vi "RTP.vi"() -> ()   [LabVIEW 2015]
uses:
  <vilib>/myRIO/Common/Instrument Driver Framework/myRIO v1.0/UART/vis/myRIO v1.0 Close UART.vi
  <vilib>/FPGAPlugInAG/myRIO-1900/niLvFpga_Open_myRIO-1900.vi
  <vilib>/rvi/interface/common/dynamic/niFpgaDynamicAddResources.vi
  <vilib>/Utility/error.llb/Error Cluster From Error Code.vi
  <vilib>/rvi/errors/niLvFpgaAdjustHostInterfaceError.vi
  <vilib>/FPGAPlugInAG/Dynamic/niLvFpga_Close_Dynamic.vi
  <vilib>/myRIO/Common/Instrument Driver Framework/Utilities/vis/FPGA Ref Manager.vi
  <vilib>/myRIO/Common/Instrument Driver Framework/myRIO v1.0/myRIO v1.0 Reset FPGA.vi
  <vilib>/myRIO/Common/Instrument Driver Framework/myRIO v1.0/IRQ/vis/myRIO v1.0 IRQ Info FGV.vi
  <vilib>/myRIO/Common/Instrument Driver Framework/myRIO v1.0/IRQ/vis/myRIO v1.0 Timer IRQ Info FGV.vi
  <vilib>/myRIO/Common/Instrument Driver Framework/myRIO v1.0/IRQ/vis/myRIO v1.0 ISR Agent.vi
  <vilib>/rvi/interface/nirviOpenFPGA/nirviOpenFPGA.xnode
  FPGA Bitfiles/adquisicion_FPGATarget_FPGA_kaZO9Kqay0w.lvbitx
  FPGA.vi
  <vilib>/rvi/interface/nirviReadWriteControl/nirviReadWriteControl.xnode
  <vilib>/rvi/interface/nirviCloseFPGA/nirviCloseFPGA.xnode
  <vilib>/rvi/interface/Simulation/niFpgaSimulationCallBeginRW.vi
  <vilib>/myRIO/Instrument Drivers/Utilities/Utilities.lvlib
  NiFpgaLv.dll
panel:
  out "Fedders current":cluster{dbl[], dbl[]}[](graph)
  out "Size":dbl
  out "u2":u16[](graph)
  out "vb":dbl
  out "vB":dbl
  out "ir":dbl
  out "i_3":dbl
  out "1_2":dbl
  out "i_1":dbl
  out "Ring":u16(ring)
  out "d 3":i16[](graph)
  out "d 2":i16[](graph)
  out "d 1":i16[](graph)
  out "i_3":u16[](graph)
  out "v_b":u16[](graph)
  out "v_B":u16[](graph)
  out "i_1":u16[](graph)
  in  "clear":bool
  in  "stop":bool
  out "State RTP":enum16{"inicio", "delay", "pedir", "guardar"}(ring)
  out "State FPGA":T1(ring)
  out "i_2":u16[](graph)
  in  "Get data":bool
  out "Data":string
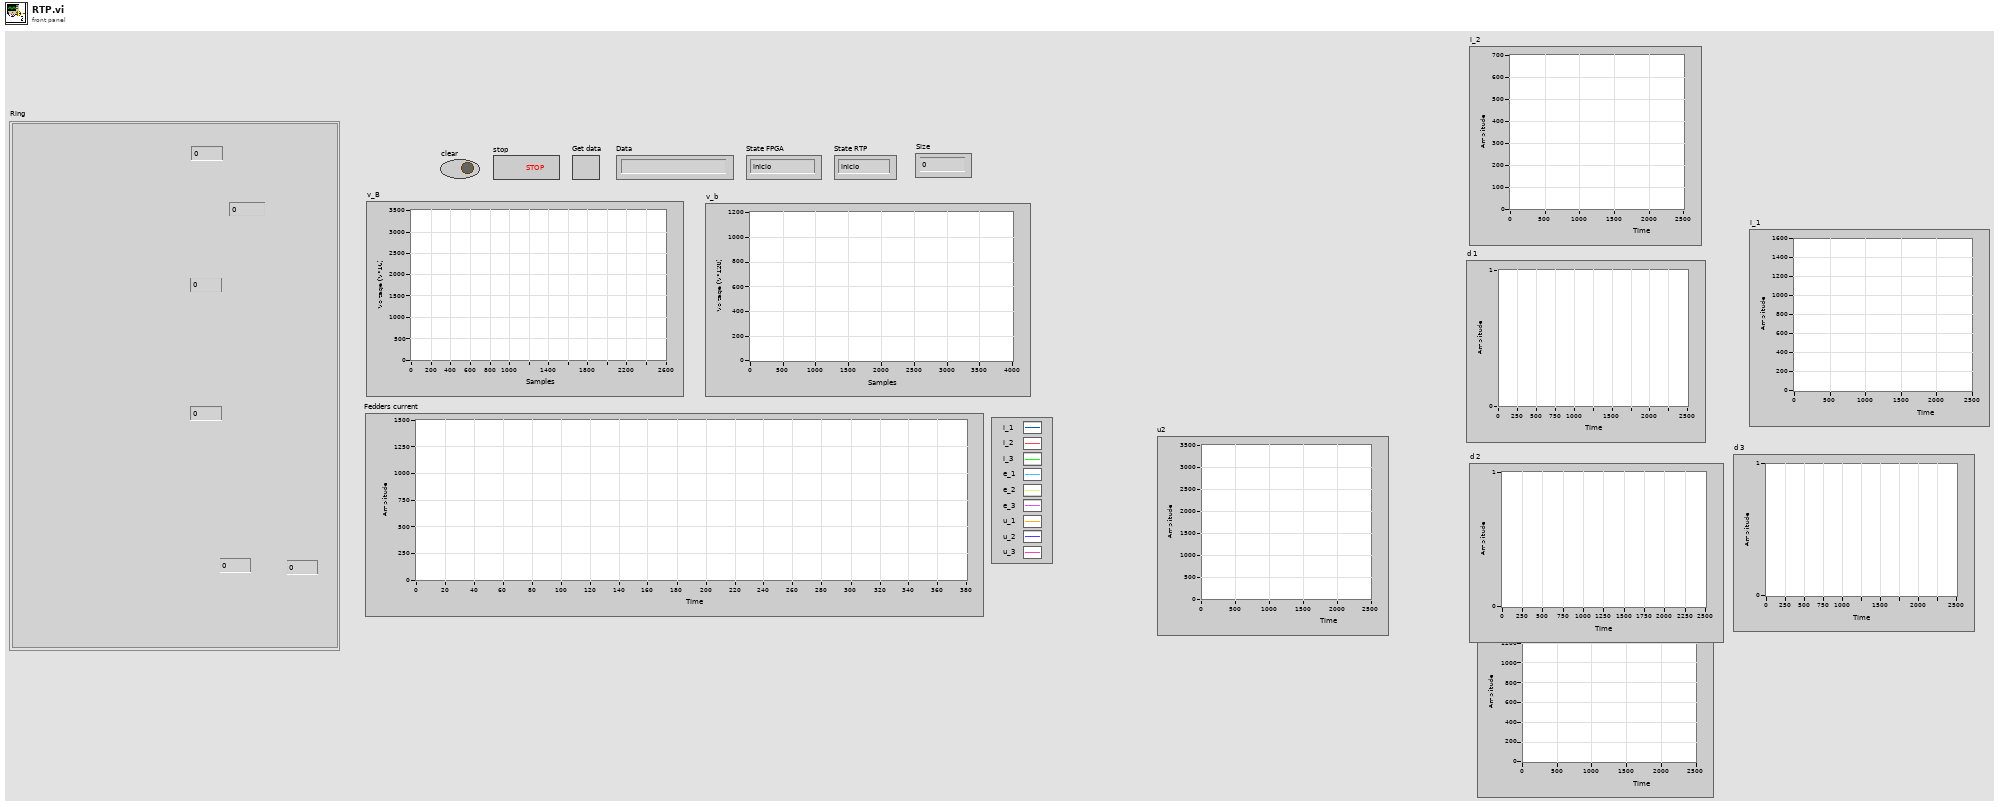
[diagram p1: front panel]
types:
  T1 = enum16{"inicio", "muestreo", "finMuestreo", "peticion", "envio"}
  T2 = cluster{u16[], u16[], u16[], u16[], u16[], i16[], i16[], i16[], u16[], u16[], u16[]}
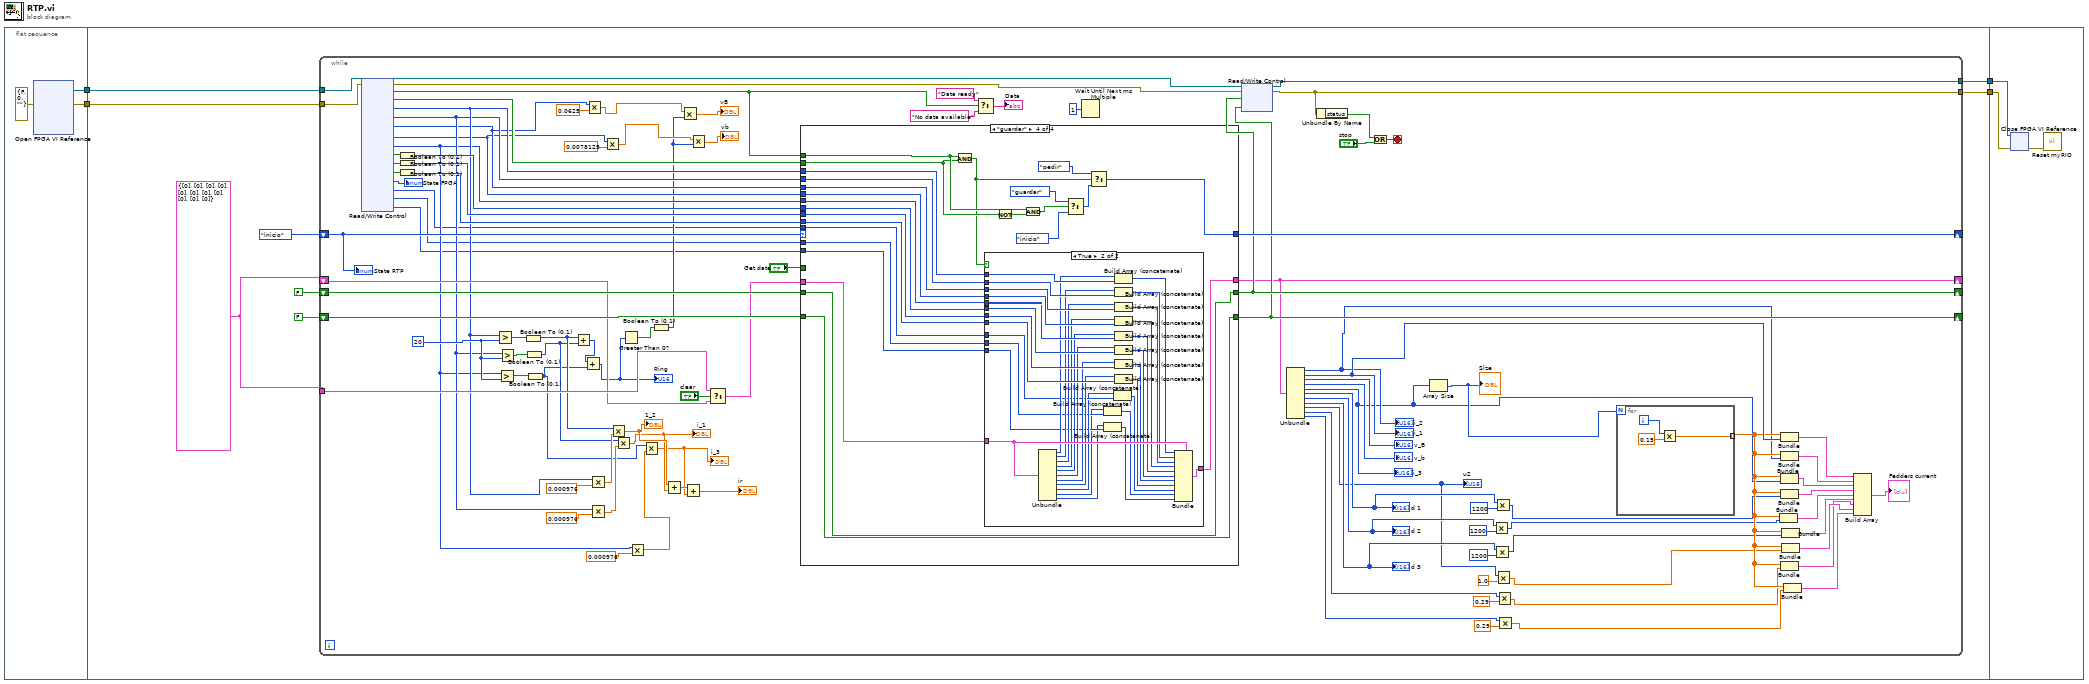
[diagram p0: block diagram]
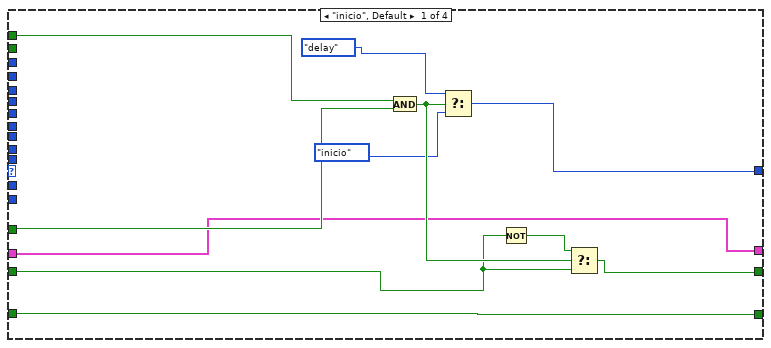
[diagram p2: hidden frame]
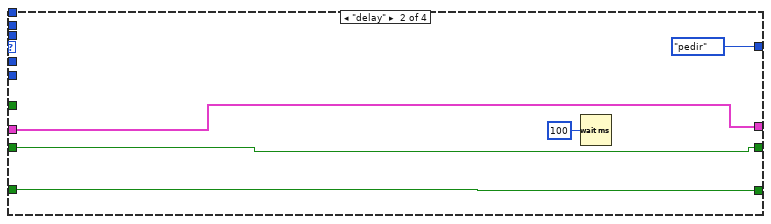
[diagram p3: hidden frame]
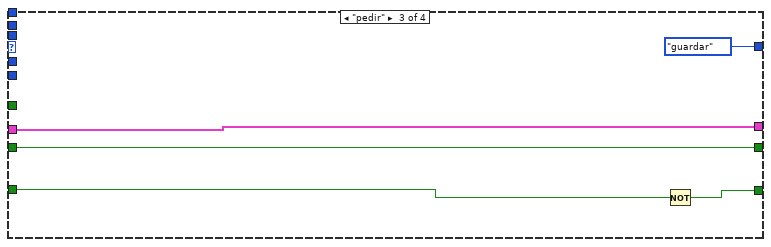
[diagram p4: hidden frame]
diagram:
  n1 = flat-sequence {
    tunnel: [w6] -> w4
    tunnel: [w5] -> w3
    tunnel: w4 -> [w15]
    tunnel: w3 -> [w14]
    tunnel: [w12] -> w2
    tunnel: [w11] -> w1
    tunnel: w2 -> [w208]
    tunnel: w1 -> [w207]
    frame #0 {
      n2 = xnode "Open FPGA VI Reference"("error in"=errorcluster {"status"=FALSE, "code"=0, "source"=""}) -> ("FPGA VI Reference Out"=w6:refnum<k20>, "error out"=w5:errorcluster)  [unwired: 1 in]
    }
    frame #1 {
      w8 = T2 {[0], [0], [0], [0], [0], [0], [0], [0], [0], [0], [0]}
      n3 = while {
        tunnel: w15 -> [w120]
        tunnel: w14 -> [w119]
        tunnel: [w109] -> w12
        tunnel: [w102] -> w11
        shift-right: [w112] -> _
        shift-left: enum16{"inicio", "delay", "pedir", "guardar"}."inicio" -> [w118]
        shift-right: [w107] -> _
        shift-left: FALSE -> [w108]
        shift-right: [w105] -> _
        shift-left: FALSE -> [w106]
        shift-right: [w87] -> _
        shift-left: w8 -> [w89]
        tunnel: w8 -> [w90]
        stop <- w100 stop-if-true
        w81 = u16 20 ("y")
        n4 = xnode "Read/Write Control"("FPGA VI Reference In"=w120, "error in"=w119) -> ("FPGA VI Reference Out"=w111:refnum<k20>, "error out"=w110:errorcluster, "ready"=w114:bool, "pased"=w104:bool, "a1"=w77:u16, "a2"=w75:u16, "a3"=w71:u16, "a4"=w69:u16, "a5"=w73:u16, "d1"=w97:bool, "d2"=w96:bool, "d3"=w95:bool, "State"=→"State FPGA":T1, "a6"=w45:u16, "a7"=w42:u16, "a8"=w41:u16)
        n5 = Boolean To (0,1)(Boolean=w97) -> (0, 1=w94:i16)
        n6 = Boolean To (0,1)(Boolean=w96) -> (0, 1=w93:i16)
        n7 = Boolean To (0,1)(Boolean=w95) -> (0, 1=w92:i16)
        n8 = Greater?(x=w77, y=w81) -> (0:w68:bool)
        n9 = Greater?(x=w73, y=w81) -> (0:w82:bool)
        n10 = Greater?(x=w75, y=w81) -> (0:w83:bool)
        n11 = Boolean To (0,1)(Boolean=w68) -> (0, 1=w67:i16)
        n12 = Boolean To (0,1)(Boolean=w83) -> (0, 1=w65:i16)
        n13 = Boolean To (0,1)(Boolean=w82) -> (0, 1=w63:i16)
        n14 = Add(x=w67, y=w65) -> (x+y=w84:i16)
        n15 = Add(x=w84, y=w63) -> (x+y=w61:i16)
        "Ring" <- w61
        n16 = Multiply(x=w71, y=0.0625) -> (x*y=w59:dbl)
        n17 = Multiply(x=w77, y=0.000976) -> (x*y=w66:dbl)
        n18 = Multiply(x=w75, y=0.000976) -> (x*y=w64:dbl)
        n19 = Multiply(x=w69, y=0.0078125) -> (x*y=w57:dbl)
        n20 = Multiply(x=w67, y=w66) -> (x*y=w54:dbl)
        "1_2" <- w54
        n21 = Multiply(x=w65, y=w64) -> (x*y=w53:dbl)
        "i_1" <- w53
        n22 = Greater Than 0?(x=w61) -> (x > 0?=w60:bool)
        n23 = Multiply(x=w73, y=0.000976) -> (x*y=w62:dbl)
        n24 = Multiply(x=w63, y=w62) -> (x*y=w52:dbl)
        "i_3" <- w52
        n25 = Boolean To (0,1)(Boolean=w60) -> (0, 1=w56:i16)
        n26 = Add(x=w54, y=w53) -> (x+y=w80:dbl)
        n27 = Multiply(x=w59, y=w56) -> (x*y=→"vB":dbl)
        n28 = Add(x=w80, y=w52) -> (x+y=→"ir":dbl)
        n29 = Multiply(x=w57, y=w56) -> (x*y=→"vb":dbl)
        n30 = Select(t=w90, s="clear", f=w89) -> (s? t:f=w88:T2)
        n31 = case shown="\"guardar\"" w118 {
          tunnel: w114 -> [w134 _ _ w165]
          tunnel: "Get data" -> [w133 _ _ _]
          tunnel: [w132 enum16{"inicio", "delay", "pedir", "guardar"}."pedir" enum16{"inicio", "delay", "pedir", "guardar"}."guardar" w168] -> w112
          tunnel: [w128 w138 w141 w158] -> w107
          tunnel: w108 -> [w129 w138 w141 w158]
          tunnel: [w125 w136 w144 w157] -> w105
          tunnel: w106 -> [w125 w136 w142 w157]
          tunnel: w104 -> [_ _ _ w164]
          tunnel: w77 -> [_ _ _ w159]
          tunnel: w75 -> [_ _ _ w154]
          tunnel: w71 -> [_ _ _ w153]
          tunnel: w69 -> [_ _ _ w152]
          tunnel: w73 -> [_ _ _ w151]
          tunnel: w94 -> [_ _ _ w150]
          tunnel: w93 -> [_ _ _ w149]
          tunnel: w92 -> [_ _ _ w148]
          tunnel: w88 -> [w124 w135 w140 w156]
          tunnel: [w124 w135 w140 w155] -> w87
          tunnel: w45 -> [_ _ _ w147]
          tunnel: w42 -> [_ _ _ w146]
          tunnel: w41 -> [_ _ _ w145]
          frame "inicio", Default {
            n32 = And(x=w134, y=w133) -> (x .and. y?=w131:bool)
            n33 = Select(t=enum16{"inicio", "delay", "pedir", "guardar"}."delay", s=w131, f=enum16{"inicio", "delay", "pedir", "guardar"}."inicio") -> (s? t:f=w132:enum16{"inicio", "delay", "pedir", "guardar"})
            n34 = Not(x=w129) -> (.not. x?=w130:bool)
            n35 = Select(t=w130, s=w131, f=w129) -> (s? t:f=w128:bool)
          }
          frame "delay" {
            n36 = Wait (ms)(milliseconds to wait=u32 100) -> ()  [unwired: 1 out]
          }
          frame "pedir" {
            n37 = Not(x=w142) -> (.not. x?=w144:bool)
          }
          frame "guardar" {
            n38 = And(x=w165, y=w164) -> (x .and. y?=w160:bool)
            n39 = case shown="True" w160 {
              tunnel: w159 -> [_ w203]
              tunnel: w156 -> [w170 w205]
              tunnel: [w170 w204] -> w155
              tunnel: w154 -> [_ w202]
              tunnel: w153 -> [_ w201]
              tunnel: w152 -> [_ w200]
              tunnel: w151 -> [_ w199]
              tunnel: w150 -> [_ w198]
              tunnel: w149 -> [_ w197]
              tunnel: w148 -> [_ w196]
              tunnel: w147 -> [_ w179]
              tunnel: w146 -> [_ w176]
              tunnel: w145 -> [_ w175]
              frame False {
              }
              frame True {
                n40 = Unbundle(w205) -> (w195:u16[], w194:u16[], w193:u16[], w192:u16[], w191:u16[], w190:i16[], w189:i16[], w188:i16[], w178:u16[], w174:u16[], w173:u16[])
                n41 = Build Array (concatenate)(w174, w176) -> (w172:u16[])
                n42 = Build Array (concatenate)(w173, w175) -> (w171:u16[])
                n43 = Build Array (concatenate)(w178, w179) -> (w177:u16[])
                n44 = Build Array (concatenate)(w195, w203) -> (w180:u16[])
                n45 = Build Array (concatenate)(w194, w202) -> (w181:u16[])
                n46 = Build Array (concatenate)(w193, w201) -> (w182:u16[])
                n47 = Build Array (concatenate)(w192, w200) -> (w183:u16[])
                n48 = Build Array (concatenate)(w191, w199) -> (w184:u16[])
                n49 = Build Array (concatenate)(w190, w198) -> (w185:i16[])
                n50 = Build Array (concatenate)(w189, w197) -> (w186:i16[])
                n51 = Build Array (concatenate)(w188, w196) -> (w187:i16[])
                n52 = Bundle(cluster=w205, w180, w181, w182, w183, w184, w185, w186, w187, w177, w172, w171) -> (w204:T2)
              }
            }
            n53 = Not(x=w164) -> (.not. x?=w166:bool)
            n54 = And(x=w165, y=w166) -> (x .and. y?=w163:bool)
            n55 = Select(t=enum16{"inicio", "delay", "pedir", "guardar"}."guardar", s=w163, f=enum16{"inicio", "delay", "pedir", "guardar"}."inicio") -> (s? t:f=w167:enum16{"inicio", "delay", "pedir", "guardar"})
            n56 = Select(t=enum16{"inicio", "delay", "pedir", "guardar"}."pedir", s=w160, f=w167) -> (s? t:f=w168:enum16{"inicio", "delay", "pedir", "guardar"})
          }
        }
        n57 = Select(t="Data ready", s=w114, f="No data available") -> (s? t:f=→"Data":string)
        n58 = Wait Until Next ms Multiple(millisecond multiple=u32 1) -> ()  [unwired: 1 out]
        n59 = xnode "Read/Write Control"("FPGA VI Reference In"=w111, "error in"=w110, "pasar"=w107, "pedir"=w105) -> ("FPGA VI Reference Out"=w109:refnum<k20>, "error out"=w102:errorcluster)
        n60 = Unbundle(w87) -> (w33:u16[], w35:u16[], →"v_B":u16[], →"v_b":u16[], w32:u16[], w48:i16[], w47:i16[], w46:i16[], w43:u16[], w38:u16[], w37:u16[])
        "i_2" <- w33
        "i_1" <- w35
        "i_3" <- w32
        "d 1" <- w48
        "d 2" <- w47
        "d 3" <- w46
        "u2" <- w43
        n61 = Unbundle By Name(w102) -> ("status"=w99:bool)
        n62 = Or(x=w99, y="stop") -> (x .or. y?=w100:bool)
        n63 = Array Size(array=w32) -> (size(s)=w36:i32)
        "Size" <- w36
        n64 = Multiply(x=w47, y=i16 1200) -> (x*y=w30:i16[])
        n65 = Multiply(x=w46, y=i16 1200) -> (x*y=w29:i16[])
        n66 = Multiply(x=w48, y=i16 1200) -> (x*y=w31:i16[])
        n67 = Multiply(x=w43, y=1.0) -> (x*y=w28:dbl[])
        n68 = Multiply(x=w38, y=0.29) -> (x*y=w27:dbl[])
        n69 = Multiply(x=w37, y=0.29) -> (x*y=w26:dbl[])
        n70 = for {
          N: w36 -> [_]
          tunnel: [w121] -> w34 mode=indexing
          i -> [w122]
          n71 = Multiply(x=w122, y=0.15) -> (x*y=w121:dbl)
        }
        n72 = Bundle(w34, w30) -> (w21:cluster{dbl[], i16[]})  [unwired: 1 in]
        n73 = Bundle(w34, w35) -> (w25:cluster{dbl[], u16[]})  [unwired: 1 in]
        n74 = Bundle(w34, w33) -> (w24:cluster{dbl[], u16[]})  [unwired: 1 in]
        n75 = Bundle(w34, w32) -> (w23:cluster{dbl[], u16[]})  [unwired: 1 in]
        n76 = Bundle(w34, w31) -> (w22:cluster{dbl[], i16[]})  [unwired: 1 in]
        n77 = Bundle(w34, w27) -> (w16:cluster{dbl[], dbl[]})  [unwired: 1 in]
        n78 = Bundle(w34, w29) -> (w20:cluster{dbl[], i16[]})  [unwired: 1 in]
        n79 = Bundle(w34, w28) -> (w17:cluster{dbl[], dbl[]})  [unwired: 1 in]
        n80 = Bundle(w34, w26) -> (w19:cluster{dbl[], dbl[]})  [unwired: 1 in]
        n81 = Build Array(w25, w24, w23, w22, w21, w20, w16, w17, w19) -> (→"Fedders current":cluster{dbl[], dbl[]}[])
        "State RTP" <- w118
      }
    }
    frame #2 {
      n82 = xnode "Close FPGA VI Reference"("FPGA VI Reference In"=w208, "error in"=w207) -> ("error out"=w206:errorcluster)
      n83 = call <vilib>:"Reset myRIO.vi"("error in (no error)"=w206) -> ()  [unwired: 10 in, 1 out]
    }
  }
